vi "Initialize OAuth for GitHub.vi"(5 "Allow Signup (T)":bool=TRUE, 7 "login":string, 9 "GitHub Access Scope":T1={"repo"=FALSE, "repo:status"=TRUE, "repo:invite"=FALSE, "repo_deployment"=FALSE, "public_repo"=TRUE, "admin:repo_hook"=FALSE, "write:repo_hook"=FALSE, "read:repo_hook"=FALSE, "admin:org"=FALSE, "write:org"=FALSE, "read:org"=FALSE, "admin:org_hook"=FALSE, "admin:public_key"=FALSE, "write:public_key"=FALSE, "read:public_key"=FALSE, "admin:gpg_key"=FALSE, "write:gpg_key"=FALSE, "read:gpg_key"=FALSE, "user"=FALSE, "read:user"=TRUE, "user:email"=FALSE, "user:follow"=FALSE, "gist"=FALSE, "notifications"=FALSE, "delete_repo"=FALSE, "write:discussion"=FALSE, "read:discussion"=TRUE, "write:packages"=FALSE, "read:packages"=TRUE, "delete:packages"=FALSE, "workflow"=FALSE, "security_events"=FALSE}, 10 "Client Secret":string, 11 "Client ID":string) -> (3 "Oauth2.GitHub":refnum<class "Oauth2.GitHub.lvclass">)   [LabVIEW 2020, in "Oauth2.GitHub.lvclass"]
uses:
  Oauth2.GitHub.lvclass
  C:/Data/1_Projects/CIGH_Oauth2/source/Oauth2/Oauth2.lvclass
  Oauth2/Oauth2.lvclass
  <vilib>/LabVIEW Open Source Project/Data Manipulation/Variant/OpenVariant.lvlib
  GitHub Access Scope -- cluster.ctl
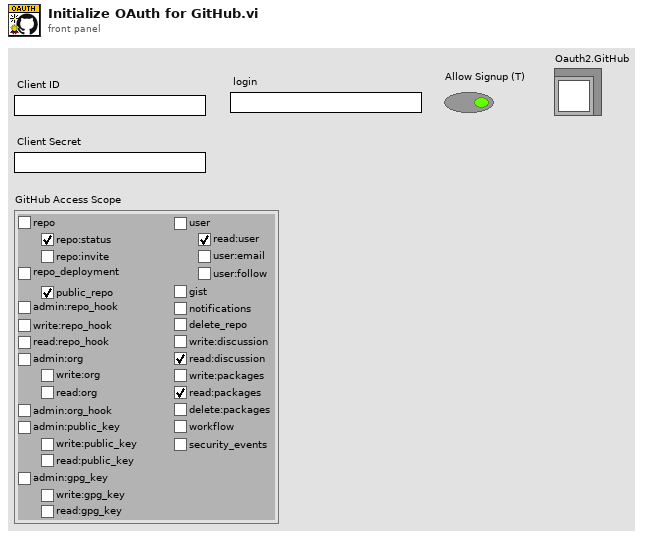
[diagram p1: front panel]
types:
  T1 = typedef "Oauth2.GitHub.lvclass/GitHub Access Scope -- cluster.ctl" = cluster{"repo":bool, "repo:status":bool, "repo:invite":bool, "repo_deployment":bool, "public_repo":bool, "admin:repo_hook":bool, "write:repo_hook":bool, "read:repo_hook":bool, "admin:org":bool, "write:org":bool, "read:org":bool, "admin:org_hook":bool, "admin:public_key":bool, "write:public_key":bool, "read:public_key":bool, "admin:gpg_key":bool, "write:gpg_key":bool, "read:gpg_key":bool, "user":bool, "read:user":bool, "user:email":bool, "user:follow":bool, "gist":bool, "notifications":bool, "delete_repo":bool, "write:discussion":bool, "read:discussion":bool, "write:packages":bool, "read:packages":bool, "delete:packages":bool, "workflow":bool, "security_events":bool}
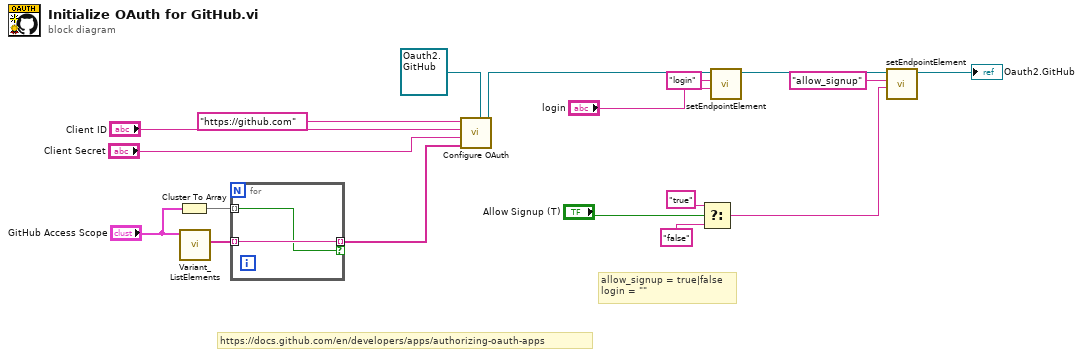
[diagram p0: block diagram]
diagram:
  # "allow_signup = true|false\t\nlogin = \"\""
  # "https://docs.github.com/en/developers/apps/authorizing-oauth-apps"
  n1 = Cluster To Array(cluster="GitHub Access Scope") -> (array=w12:bool[])
  n2 = call <vilib>:"Variant_ListElements.vi"("Variant"="GitHub Access Scope") -> ("element names"=w13:string[])  [unwired: 7 in, 3 out]
  n3 = for {
    tunnel: [w20] -> w11 mode=indexing if=w19
    tunnel: w13 -> [w20] mode=indexing
    tunnel: w12 -> [w19] mode=indexing
  }
  n4 = call "Configure OAuth.vi"("Oauth2 in"=refnum<class "Oauth2.GitHub.lvclass"> refnum ("Oauth2.GitHub in"), "scopes"=w11, "Client Secret"="Client Secret", "Client ID"="Client ID", "Authorization Server URI"="https://github.com") -> ("Oauth2"=w9:refnum<class "Oauth2.GitHub.lvclass">)  [unwired: 5 in, 1 out]
  n5 = Select(t="true" ("Endpoint Name"), s="Allow Signup (T)", f="false" ("Endpoint Name")) -> (s? t:f=w1:string)
  n6 = call "setEndpointElement.vi"("Value"="login", "Endpoint Name"="login", "Oauth2 in"=w9) -> ("Oauth2 out"=w10:refnum<class "Oauth2.GitHub.lvclass">)  [unwired: 7 in, 1 out]
  n7 = call "setEndpointElement.vi"("Value"=w1, "Endpoint Name"="allow_signup", "Oauth2 in"=w10) -> ("Oauth2 out"=→"Oauth2.GitHub":refnum<class "Oauth2.GitHub.lvclass">)  [unwired: 7 in, 1 out]
